vi "Calibrate Camera.vi"(5 "Termination Criteria (Default: Default Criteria) in":refnum<class "Termination Criteria.lvclass">, 6 "Camera Parameters (Estimate)":T13, 7 "Flags (Default: Empty)":T4[](array[typedef]), 8 "error in (no error)":errorcluster, 9 "Fixed Point Index (Default -1: Do not use RO mode)":i32=-1, 10 "Image Size":T12, 11 "Point Correspondences":T5) -> (0 "error out":errorcluster, 1 "RMS Error":dbl[](array[numeric]), 3 "Camera Parameters":T9, 4 "Poses":T1[](array[typedef]))   [LabVIEW 2020, in "ar.lvlib"]
doc: "Compute the Camera Calibration based on the point correspondences.\n\nInternally this VI wraps the OpenCV CalibrateCameraRO function which is documented at https://docs.opencv.org/4.10.0/d9/d0c/group__calib3d.html#ga11eeb16e5a458e1ed382fb27f585b753"
uses:
  ar.lvlib
  Camera Parameters Estimate.ctl
  common/Camera Matrix.ctl
  common/Camera Distortion Coefficients.ctl
  common/Image Size (Integer).ctl
  common/Camera Parameters.ctl
  Point Correspondence Sets.ctl
  Point Correspondence Set.ctl
  common/Object Point (Float).ctl
  common/Image Point (Float).ctl
  Camera Calibration Flags.ctl
  common/Termination Criteria/Termination Criteria.lvclass
  Pose.ctl
  rvec.ctl
  tvec.ctl
  common/Termination Criteria/Termination Criteria.lvclass/Termination Criteria.ctl
  common/common.lvlib
  common/bin/gartoolkit_ar_32-1.dll
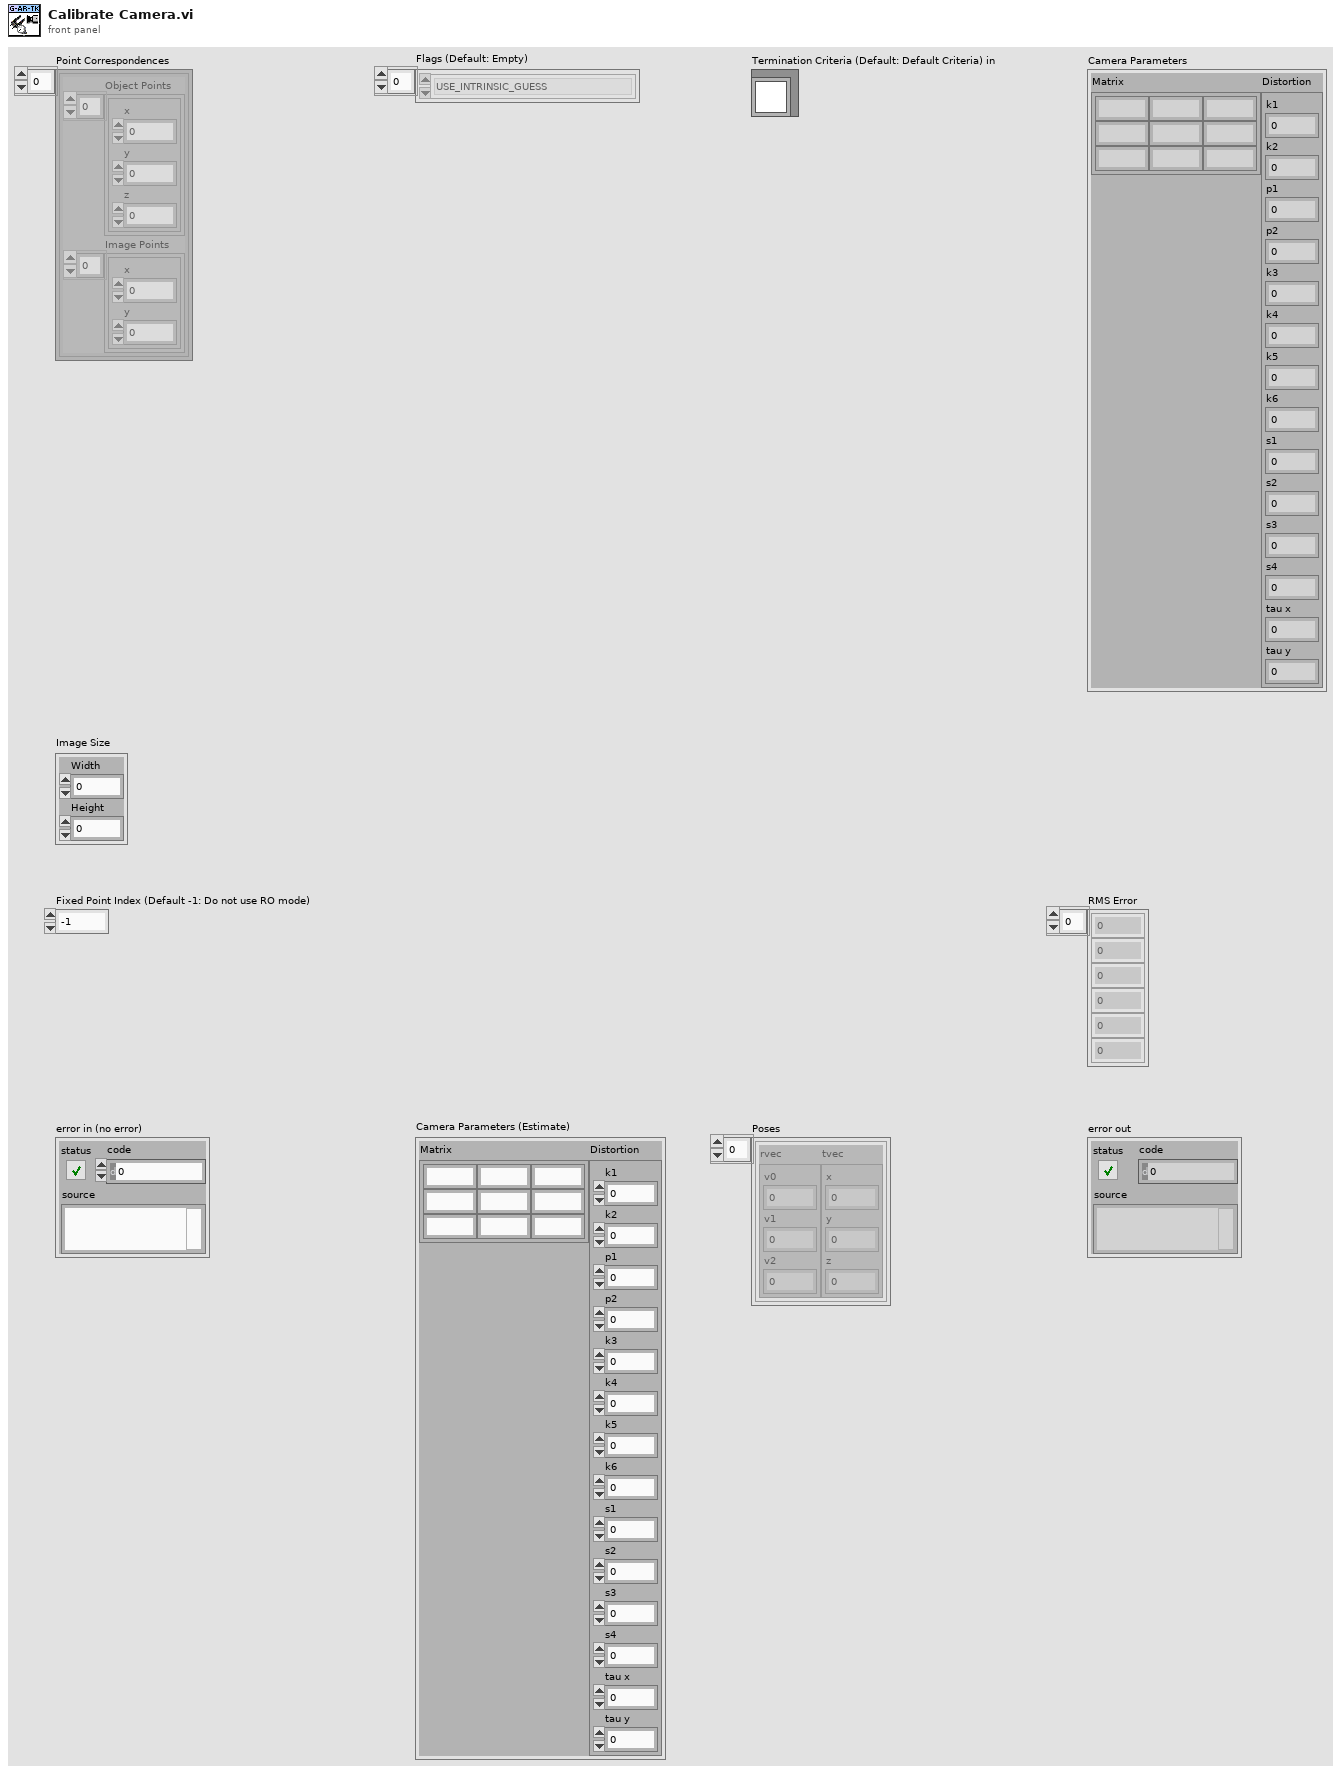
[diagram p1: front panel]
types:
  T1 = typedef "ar.lvlib/Pose.ctl" = cluster{"rvec":T2, "tvec":T3}
  T2 = typedef "ar.lvlib/rvec.ctl" = cluster{"v0":dbl, "v1":dbl, "v2":dbl}
  T3 = typedef "ar.lvlib/tvec.ctl" = cluster{"x":dbl, "y":dbl, "z":dbl}
  T4 = typedef "ar.lvlib/Camera Calibration Flags.ctl" = enum16{"USE_INTRINSIC_GUESS", "FIX_PRINCIPAL_POINT", "FIX_ASPECT_RATIO", "ZERO_TANGENT_DIST", "FIX_FOCAL_LENGTH", "FIX_K1", "RATIONAL_MODEL", "THIN_PRISM_MODEL", "FIX_S1_S2_S3_S4", "TILTED_MODEL", "FIX_TAUX_TAUY"}
  T5 = typedef "ar.lvlib/Point Correspondence Sets.ctl" = T6[]
  T6 = typedef "ar.lvlib/Point Correspondence Set.ctl" = cluster{"Object Points":T7[], "Image Points":T8[]}
  T7 = typedef "common.lvlib/Object Point (Float).ctl" = cluster{"x":dbl, "y":dbl, "z":dbl}
  T8 = typedef "common.lvlib/Image Point (Float).ctl" = cluster{"x":dbl, "y":dbl}
  T9 = typedef "common.lvlib/Camera Parameters.ctl" = cluster{"Matrix":T10, "Distortion":T11}
  T10 = typedef "common.lvlib/Camera Matrix.ctl" = cluster{"m 0,0":dbl, "m 0,1":dbl, "m 0,2":dbl, "m 1,0":dbl, "m 1,1":dbl, "m 1,2":dbl, "m 2,0":dbl, "m 2,1":dbl, "m 2,2":dbl}
  T11 = typedef "common.lvlib/Camera Distortion Coefficients.ctl" = cluster{"k1":dbl, "k2":dbl, "p1":dbl, "p2":dbl, "k3":dbl, "k4":dbl, "k5":dbl, "k6":dbl, "s1":dbl, "s2":dbl, "s3":dbl, "s4":dbl, "tau x":dbl, "tau y":dbl}
  T12 = typedef "common.lvlib/Image Size (Integer).ctl" = cluster{"Width":u16, "Height":u16}
  T13 = typedef "ar.lvlib/Camera Parameters Estimate.ctl" = cluster{"Matrix":T10, "Distortion":T11}
  T14 = typedef "common.lvlib/Termination Criteria.lvclass/Termination Criteria Values.ctl" = cluster{"Epsilon":dbl, "Iterations":i32}
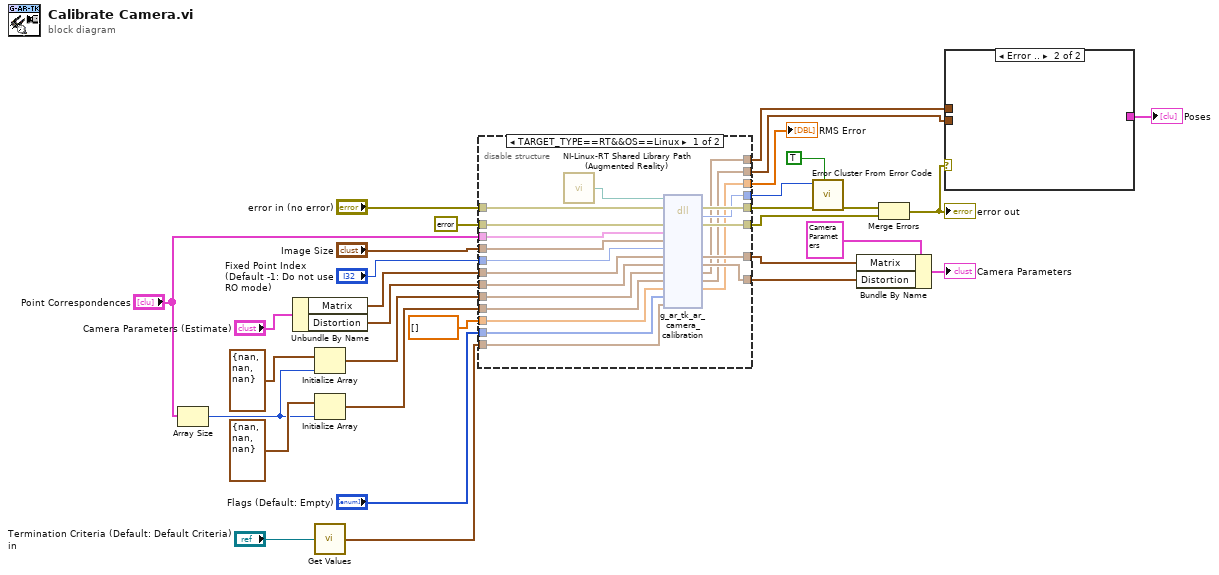
[diagram p0: block diagram]
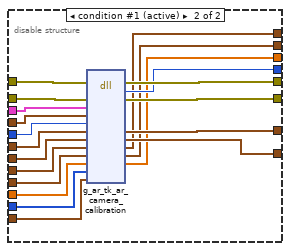
[diagram p2: hidden frame]
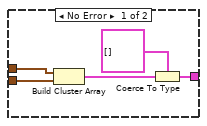
[diagram p3: hidden frame]
diagram:
  n1 = Array Size(array="Point Correspondences") -> (size(s)=w26:i32)
  n2 = Unbundle By Name("Camera Parameters (Estimate)") -> ("Matrix"=w16:T10, "Distortion"=w15:T11)
  n3 = Initialize Array(T2 {"v0"=nan, "v1"=nan, "v2"=nan} ("rvec"), w26) -> (w14:T2[])
  n4 = Initialize Array(T3 {"x"=nan, "y"=nan, "z"=nan} ("tvec"), w26) -> (w13:T3[])
  n5 = call "Get Values.vi"("Termination Criteria in"="Termination Criteria (Default: Default Criteria) in") -> ("Term Criteria"=w10:T14)
  n6 = disable-structure shown="TARGET_TYPE==RT&&OS==Linux" {
    disable-tunnel: "error in (no error)" -> [w51 w72]
    disable-tunnel: errorcluster {"status"=FALSE, "code"=0, "source"=""} ("error constant") -> [w50 w71]
    disable-tunnel: "Point Correspondences" -> [w49 w70]
    disable-tunnel: "Image Size" -> [w48 w69]
    disable-tunnel: "Fixed Point Index (Default -1: Do not use RO mode)" -> [w47 w68]
    disable-tunnel: w16 -> [w46 w67]
    disable-tunnel: w15 -> [w45 w66]
    disable-tunnel: w14 -> [w44 w65]
    disable-tunnel: w13 -> [w43 w64]
    disable-tunnel: dbl[] [] ("rms_errors") -> [w42 w63]
    disable-tunnel: "Flags (Default: Empty)" -> [w41 w62]
    disable-tunnel: w10 -> [w40 w61]
    disable-tunnel: [w39 w60] -> w9
    disable-tunnel: [w38 w59] -> w8
    disable-tunnel: [w37 w58] -> w7
    disable-tunnel: [w36 w57] -> w6
    disable-tunnel: [w35 w56] -> w5
    disable-tunnel: [w34 w55] -> w4
    disable-tunnel: [w33 w54] -> w3
    disable-tunnel: [w32 w53] -> w2
    frame condition #0 {
      n7 = call "NI-Linux-RT Shared Library Path (Augmented Reality).vi"() -> ("Path"=w52:path)
      n8 = dll-call lib="?" fn="g_ar_tk_ar_camera_calibration" ("g_ar_toolkit.*.*:g_ar_tk_image_copy")(path in=w52, error in=w51, "error_cluster"=w50, "corespondences"=w49, "image_size"=w48, "fixed_point"=w47, "camera_matrix"=w46, "camera_distortion"=w45, "rvecs"=w44, "tvecs"=w43, "rms_errors"=w42, "flags"=w41, "termination_crit"=w40) -> (error out=w39:errorcluster, w38:i32, "error_cluster"=w37:errorcluster, "camera_matrix"=w36:T10, "camera_distortion"=w35:T11, "rvecs"=w34:T2[], "tvecs"=w33:T3[], "rms_errors"=w32:dbl[])  [unwired: 6 in, 1 out]
    }
    frame condition #1 (active) {
      n9 = dll-call lib="C:/serenial/lib/g-augmented-reality-toolkit/LabVIEW/common/bin/gartoolkit_ar_*-1.*" fn="g_ar_tk_ar_camera_calibration" ("g_ar_toolkit.*.*:g_ar_tk_image_copy")(error in=w72, "error_cluster"=w71, "corespondences"=w70, "image_size"=w69, "fixed_point"=w68, "camera_matrix"=w67, "camera_distortion"=w66, "rvecs"=w65, "tvecs"=w64, "rms_errors"=w63, "flags"=w62, "termination_crit"=w61) -> (error out=w60:errorcluster, w59:i32, "error_cluster"=w58:errorcluster, "camera_matrix"=w57:T10, "camera_distortion"=w56:T11, "rvecs"=w55:T2[], "tvecs"=w54:T3[], "rms_errors"=w53:dbl[])  [unwired: 7 in, 1 out]
    }
  }
  "RMS Error" <- w2
  n10 = call <vilib>:"Error Cluster From Error Code.vi"("show call chain? (False)"=TRUE, "error in (no error)"=w9, "error code (0)"=w8) -> ("error out"=w31:errorcluster)  [unwired: 6 in]
  n11 = Bundle By Name(cluster=T9 {"Matrix"={"m 0,0"=0.0, "m 0,1"=0.0, "m 0,2"=0.0, "m 1,0"=0.0, "m 1,1"=0.0, "m 1,2"=0.0, "m 2,0"=0.0, "m 2,1"=0.0, "m 2,2"=0.0}, "Distortion"={"k1"=0.0, "k2"=0.0, "p1"=0.0, "p2"=0.0, "k3"=0.0, "k4"=0.0, "k5"=0.0, "k6"=0.0, "s1"=0.0, "s2"=0.0, "s3"=0.0, "s4"=0.0, "tau x"=0.0, "tau y"=0.0}} ("Camera Parameters"), "Matrix"=w6, "Distortion"=w5) -> (→"Camera Parameters":T9)
  n12 = Merge Errors(w31, w7) -> (w25:errorcluster)
  "error out" <- w25
  n13 = case shown="Error .." w25 {
    tunnel: w4 -> [w77 _]
    tunnel: w3 -> [w76 _]
    tunnel: [w73 _] -> w27
    frame No Error {
      n14 = Build Cluster Array(w77, w76) -> (w74:cluster{"rvec":T2, "tvec":T3}[])
      n15 = Coerce To Type(0:w74, 1:T1[] [] ("Array")) -> (2:w73:T1[])
    }
    frame Error {
    }
  }
  "Poses" <- w27
